vi "Get Scope Error Files Properties.vi"(7 "scope":T2, 8 "error in (no error)":errorcluster, 11 "error list <top>":variant) -> (0 "error out":errorcluster, 1 "simplified paths":string[](array[string]), 2 "properties":T1[](array[typedef]), 3 "error list <top> dup":variant, 4 "parsable":bool[](array[boolean]))   [LabVIEW 2017]
uses:
  Scope.ctl
  Error Code File Properties.ctl
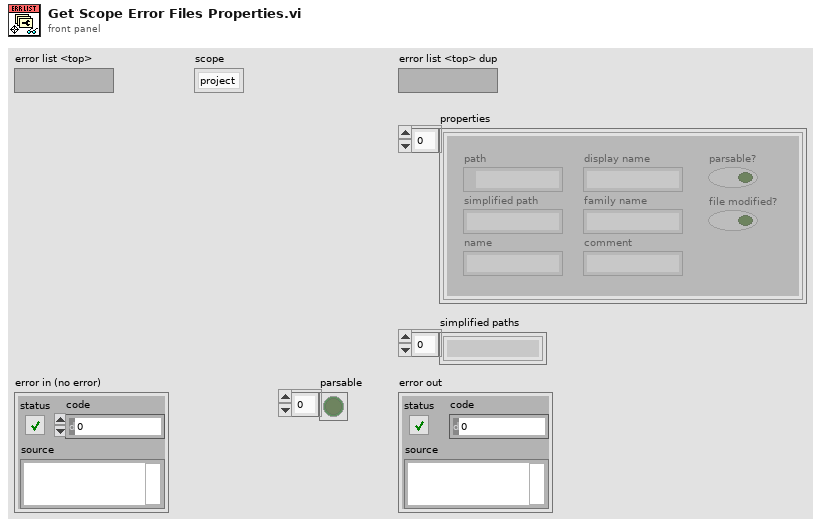
[diagram p1: front panel]
types:
  T1 = typedef "Error Code File Properties.ctl" = cluster{"path":path, "simplified path":string, "name":string, "display name":string, "family name":string, "comment":string, "parsable?":bool, "file modified?":bool}
  T2 = typedef "Scope.ctl" = enum16{"project", "global"}
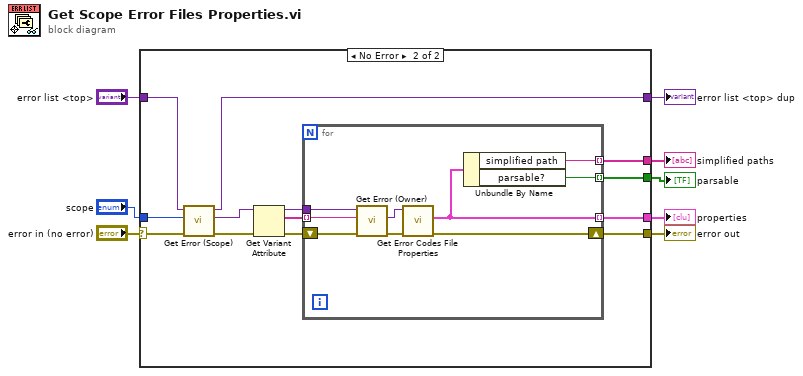
[diagram p0: block diagram]
diagram:
  n1 = case shown="No Error" "error in (no error)" {
    selector: "error in (no error)" -> [w10 w16]
    tunnel: "scope" -> [_ w23]
    tunnel: [w10 w17] -> w6
    tunnel: "error list <top>" -> [w9 w15]
    tunnel: [w9 w14] -> w4
    tunnel: [_ w13] -> w3
    tunnel: [_ w12] -> w2
    tunnel: [_ w11] -> w1
    frame Error {
    }
    frame No Error {
      n2 = call "Get Error (Scope).vi"("error in (no error)"=w16, "scope"=w23, "error list <top>"=w15) -> ("error out"=w18:errorcluster, "error list <scope>"=w20:variant, "error list <top> dup"=w14:variant)  [unwired: 5 in, 1 out]
      n3 = Get Variant Attribute(Variant=w20, error in=w18) -> (duplicate Variant=w21:variant, names=w22:string[], error out=w19:errorcluster)  [unwired: 2 in, 1 out]
      n4 = for {
        shift-right: [w26] -> w17
        shift-left: w19 -> [w32]
        tunnel: w22 -> [w30] mode=indexing
        tunnel: w21 -> [w31]
        tunnel: [w25] -> w13 mode=indexing
        tunnel: [w29] -> w12 mode=indexing
        tunnel: [w28] -> w11 mode=indexing
        n5 = call "Get Error (Owner).vi"("error in (no error)"=w32, "owner"=w30, "error list <scope>"=w31) -> ("error out"=w27:errorcluster, "error list <owner>"=w24:variant)  [unwired: 5 in, 2 out]
        n6 = call "Get Error Codes File Properties.vi"("error in (no error)"=w27, "error list <owner> in"=w24) -> ("error out"=w26:errorcluster, "properties"=w25:T1)  [unwired: 6 in, 2 out]
        n7 = Unbundle By Name(w25) -> ("simplified path"=w29:string, "parsable?"=w28:bool)
      }
    }
  }
  "error out" <- w6
  "error list <top> dup" <- w4
  "properties" <- w3
  "simplified paths" <- w2
  "parsable" <- w1
